vi "Keithley 2002 RTD Config.vi"(0 "GPIB address":string="16", 1 "reference (off:0)":u16(ring) items=["off", "set reference value"], 2 "reference value (degs)":dbl format="%^.2e", 3 "transducer (2-W RTD-PT385:0)":u16(ring) items=["2-wire RTD - PT385", "2-wire RTD - PT3916", "2-wire RTD - USER", "2-wire RTD - F100", "2-wire RTD - D100", "2-wire RTD - PT100", "4-wire RTD - PT385", "4-wire RTD - PT3916", "4-wire RTD - USER", "4-wire RTD - F100", "4-wire RTD - D100", "4-wire RTD - PT100"], 4 "alpha":dbl=0.00385 min=0.0 max=0.01 format="%^.5e", 5 "integration time (0:auto)":u16(ring) items=["automatic", "automatic once", "set to minimum", "set to maximum", "set aperature value", "set NPLC value"], 6 "beta":dbl=0.111 min=0.0 max=1.0 format="%^.5e", 7 "integ. value":dbl=0.01667 format="%^.2e", 8 "delta":dbl=1.507 min=0.0 max=5.0 format="%^.5e", 9 "resolution (5.5 digits:4)":u16(ring)=4 items=["auto resolution", "auto resolution once", "3.5 digits", "4.5 digits", "5.5 digits", "6.5 digits"], 10 "Rzero":dbl=100.0 min=0.0 max=1000.0 format="%^.5e", 11 "error in":T1, 12 "digital filter (off:0)":u16(ring) items=["off", "auto filter", "auto filter once", "moving filter", "repeating filter"], 13 "dig. filter count":dbl=10.0 min=1.0 max=100.0 step=1.0 format="%^.2e", 14 "temp (celsius:0)":u16(ring) items=["Celsius", "Fahrenheit", "Kelvin"]) -> (15 "error out":T1)   [LabVIEW 2020]
doc: "This VI is used to configure the settings for the RTD temperature measurements. The instrument can be in any mode when this VI is run. The settings will go into effect and the instrument will go into the Temperature mode."
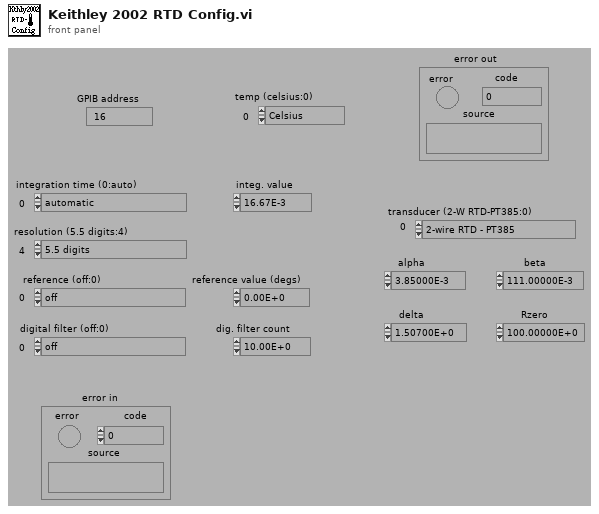
[diagram p1: front panel]
types:
  T1 = cluster{"error":bool, "code":i32, "source":string}
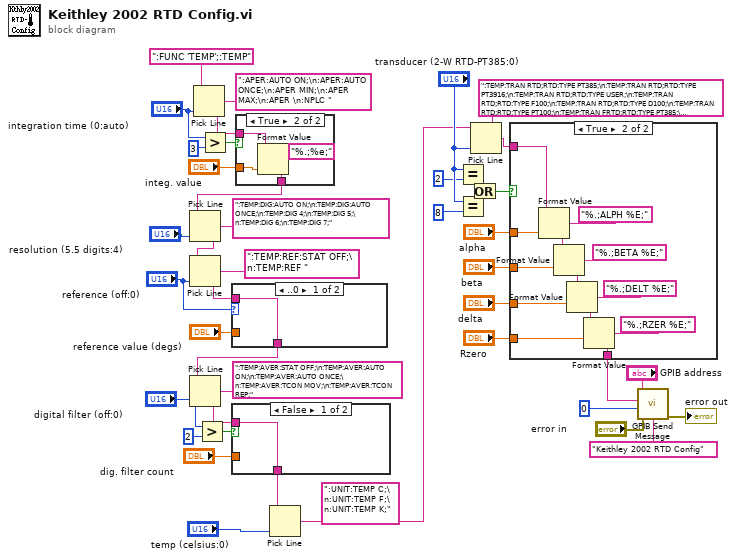
[diagram p0: block diagram]
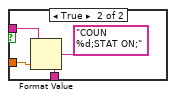
[diagram p3: hidden frame]
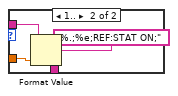
[diagram p4: hidden frame]
diagram:
  n1 = Pick Line(string ("")=":FUNC 'TEMP';:TEMP", multi-line string=":APER:AUTO ON;\n:APER:AUTO ONCE;\n:APER MIN;\n:APER MAX;\n:APER \n:NPLC ", line index="integration time (0:auto)") -> (output string=w38:string)
  n2 = Greater?(x="digital filter (off:0)", y=2) -> (0:w26:bool)
  n3 = Greater?(x="integration time (0:auto)", y=3) -> (0:w39:bool)
  n4 = case shown="True" w39 {
    tunnel: "integ. value" -> [_ w48]
    tunnel: w38 -> [w45 w47]
    tunnel: [w45 w46] -> w18
    frame False {
    }
    frame True {
      n5 = Format Value(string ("")=w47, format string="%.;%e;", value (0)=w48) -> (output string=w46:string)
    }
  }
  n6 = Pick Line(string ("")=w18, multi-line string=":TEMP:DIG:AUTO ON;\n:TEMP:DIG:AUTO ONCE;\n:TEMP:DIG 4;\n:TEMP:DIG 5;\n:TEMP:DIG 6;\n:TEMP:DIG 7;", line index="resolution (5.5 digits:4)") -> (output string=w32:string)
  n7 = Pick Line(string ("")=w32, multi-line string=":TEMP:REF:STAT OFF;\n:TEMP:REF ", line index="reference (off:0)") -> (output string=w35:string)
  n8 = case shown="..0" "reference (off:0)" {
    tunnel: "reference value (degs)" -> [_ w54]
    tunnel: w35 -> [w50 w53]
    tunnel: [w50 w51] -> w19
    frame ..0 {
    }
    frame 1.. {
      n9 = Format Value(string ("")=w53, format string="%.;%e;REF:STAT ON;", value (0)=w54) -> (output string=w51:string)
    }
  }
  n10 = Pick Line(string ("")=w19, multi-line string=":TEMP:AVER:STAT OFF;\n:TEMP:AVER:AUTO ON;\n:TEMP:AVER:AUTO ONCE;\n:TEMP:AVER:TCON MOV;\n:TEMP:AVER:TCON REP;", line index="digital filter (off:0)") -> (output string=w29:string)
  n11 = case shown="False" w26 {
    tunnel: "dig. filter count" -> [_ w59]
    tunnel: w29 -> [w55 w58]
    tunnel: [w55 w57] -> w3
    frame False {
    }
    frame True {
      n12 = Format Value(string ("")=w58, format string="COUN %d;STAT ON;", value (0)=w59) -> (output string=w57:string)
    }
  }
  n13 = Pick Line(string ("")=w3, multi-line string=":UNIT:TEMP C;\n:UNIT:TEMP F;\n:UNIT:TEMP K;", line index="temp (celsius:0)") -> (output string=w1:string)
  n14 = Equal?(x="transducer (2-W RTD-PT385:0)", y=2) -> (x = y?=w6:bool)
  n15 = Equal?(x="transducer (2-W RTD-PT385:0)", y=8) -> (x = y?=w5:bool)
  n16 = Or(x=w6, y=w5) -> (x .or. y?=w13:bool)
  n17 = Pick Line(string ("")=w1, multi-line string=":TEMP:TRAN RTD;RTD:TYPE PT385;\n:TEMP:TRAN RTD;RTD:TYPE PT3916;\n:TEMP:TRAN RTD;RTD:TYPE USER;\n:TEMP:TRAN RTD;RTD:TYPE F100;\n:TEMP:TRAN RTD;RTD:TYPE D100;\n:TEMP:TRAN RTD;RTD:TYPE PT100;\n:TEMP:TRAN FRTD;RTD:TYPE PT385;\n:TEMP:TRAN FRTD;RTD:TYPE PT3916;\n:TEMP:TRAN FRTD;RTD:TYPE USER;\n:TEMP:TRAN FRTD;RTD:TYPE F100;\n:TEMP:TRAN FRTD;RTD:TYPE D100;\n:TEMP:TRAN FRTD;RTD:TYPE PT100;", line index="transducer (2-W RTD-PT385:0)") -> (output string=w8:string)
  n18 = case shown="True" w13 {
    tunnel: "alpha" -> [_ w69]
    tunnel: "beta" -> [_ w68]
    tunnel: "delta" -> [_ w67]
    tunnel: "Rzero" -> [_ w66]
    tunnel: w8 -> [w60 w65]
    tunnel: [w60 w61] -> w7
    frame False {
    }
    frame True {
      n19 = Format Value(string ("")=w65, format string="%.;ALPH %E;", value (0)=w69) -> (output string=w64:string)
      n20 = Format Value(string ("")=w64, format string="%.;BETA %E;", value (0)=w68) -> (output string=w63:string)
      n21 = Format Value(string ("")=w63, format string="%.;DELT %E;", value (0)=w67) -> (output string=w62:string)
      n22 = Format Value(string ("")=w62, format string="%.;RZER %E;", value (0)=w66) -> (output string=w61:string)
    }
  }
  n23 = call "GPIB Send Message.vi"("address string"="GPIB address", "write buffer"=w7, "source"="Keithley 2002 RTD Config", "write mode (set END:0)"=0, "error in"="error in") -> ("error out"=→"error out":T1)  [unwired: 2 in, 2 out]
